vi "Get Measurement Frequency.vi"() -> (2 "Measurments per hour":dbl, 3 "Seconds":dbl)   [LabVIEW 2017, in "Akwizycja.lvlib"]
uses:
  Akwizycja.lvlib
  <vilib>/Utility/config.llb/NI_LVConfig.lvlib
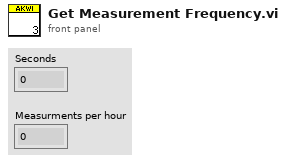
[diagram p1: front panel]
types:
  T1 = typedef "NI_LVConfig.lvlib/Config Data RefNum.ctl" = refnum<k1>
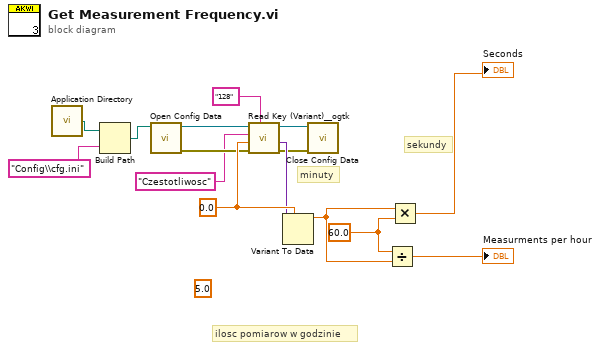
[diagram p0: block diagram]
diagram:
  (unwired) 5.0
  w14 = 0.0
  w15 = 60.0
  # "ilosc pomiarow w godzinie"
  # "sekundy"
  # "minuty"
  n1 = call <vilib>:"Application Directory.vi"() -> ("Application Directory"=w1:path)
  n2 = Build Path(base path=w1, name or relative path="Config\\cfg.ini") -> (appended path=w3:path)
  n3 = call <vilib>:"Open Config Data.vi"("configuration file path"=w3) -> ("error out"=w7:errorcluster, "refnum"=w4:T1)  [unwired: 8 in, 1 out]
  n4 = call <userlib>:"Read Key (Variant)__ogtk.vi"("section"="128", "error in (no error)"=w7, "type"=w14, "key (optional)"="Czestotliwosc", "refnum"=w4) -> ("error out"=w8:errorcluster, "key-value"=w9:variant, "refnum out"=w10:T1)  [unwired: 3 in, 1 out]
  n5 = Variant To Data(type=w14, Variant=w9) -> (data=w12:dbl)  [unwired: 1 in, 1 out]
  n6 = call <vilib>:"Close Config Data.vi"("error in (no error)"=w8, "refnum"=w10) -> ()  [unwired: 8 in, 2 out]
  n7 = Divide(x=w15, y=w12) -> (x/y=→"Measurments per hour":dbl)
  n8 = Multiply(x=w12, y=w15) -> (x*y=→"Seconds":dbl)
